vi "FringeScannerCloseSynchronization.vi"(2 "FringeTrackerSynchro":T1, 9 "error in (no error)":errorcluster) -> (6 "error out":errorcluster)   [LabVIEW 2009]
uses:
  Controls/FringeTrackerSynchro.ctl
  Controls/FringeScannerCommand.ctl
  Controls/FringeScannerData.ctl
  Nicmos/Controls/NICMOS.READOUT.ctl
  Controls/FringeScannerState.ctl
  Controls/FringeScannerInfo.ctl
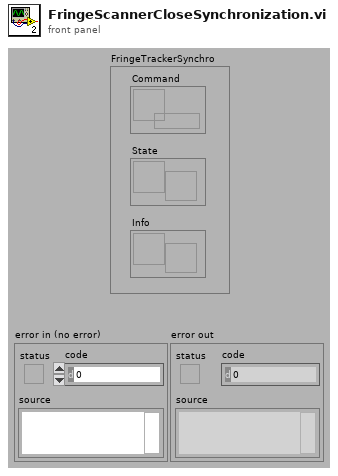
[diagram p1: front panel]
types:
  T1 = typedef "FringeTrackerSynchro.ctl" = cluster{"Command":refnum<queue>, "State":refnum<notifier>, "Info":refnum<notifier>}
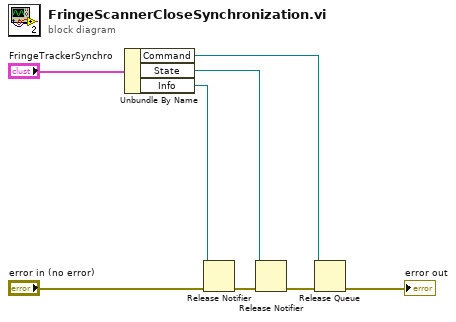
[diagram p0: block diagram]
diagram:
  n1 = Unbundle By Name("FringeTrackerSynchro") -> ("Command"=w6:refnum<queue>, "State"=w7:refnum<notifier>, "Info"=w1:refnum<notifier>)
  n2 = Release Notifier(notifier=w1, error in (no error)="error in (no error)") -> (error out=w2:errorcluster)  [unwired: 1 in, 2 out]
  n3 = Release Notifier(notifier=w7, error in (no error)=w2) -> (error out=w5:errorcluster)  [unwired: 1 in, 2 out]
  n4 = Release Queue(queue=w6, error in (no error)=w5) -> (error out=→"error out":errorcluster)  [unwired: 1 in, 2 out]
